vi "Run Test Suite.vi"(8 "error in (no error)":errorcluster, 10 "Test Suite In":refnum<class "LUnit Test Suite.lvclass">, 11 "Test Runner In":refnum<class "Test Runner.lvclass">) -> (0 "error out":errorcluster, 3 "Test Runner Out":refnum<class "Test Runner.lvclass">)   [LabVIEW 2020, in "Test Runner.lvclass"]
uses:
  Test Runner.lvclass
  C:/Git/astemes-lunit/source/Application Framework/Process Classes/Process/Process.lvclass
  Test Suite/LUnit Test Suite.lvclass
  Application Framework/Process Classes/Process/Process.lvclass/Process.ctl
  Application Framework/Process Classes/Process/Process.lvclass
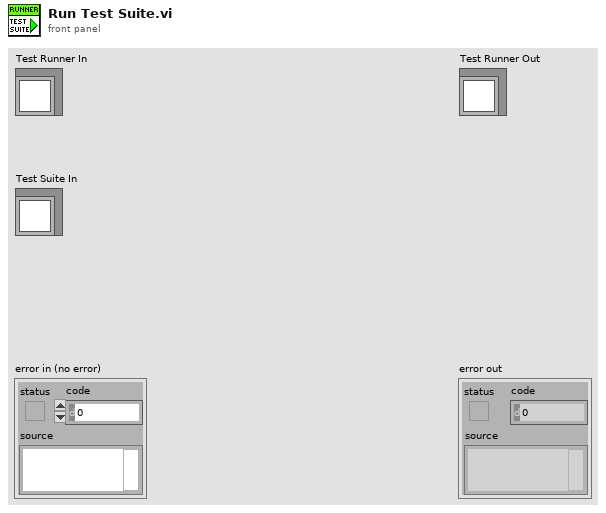
[diagram p1: front panel]
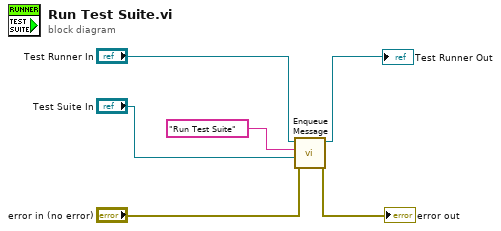
[diagram p0: block diagram]
diagram:
  n1 = call "Enqueue Message.vi"("error in (no error)"="error in (no error)", "Message Data"="Test Suite In", "Message"="Run Test Suite", "Process In"="Test Runner In") -> ("error out"=→"error out":errorcluster, "Process Out"=→"Test Runner Out":refnum<class "Test Runner.lvclass">)  [unwired: 6 in]
